vi "readFrequencySweep(sub).vi"(0 "resourcein":refnum<visa-resource-name>, 1 "Command":dbl, 2 "Commandprefix":string="R0003", 3 "errorin":errorcluster, 4 "Numeric":i32) -> (5 "resourceout":refnum<visa-resource-name>, 6 "Array":string[](array[string]), 7 "errorout":errorcluster)   [LabVIEW 2015]
panel:
  out "output 2":string
  out "output 1":dbl
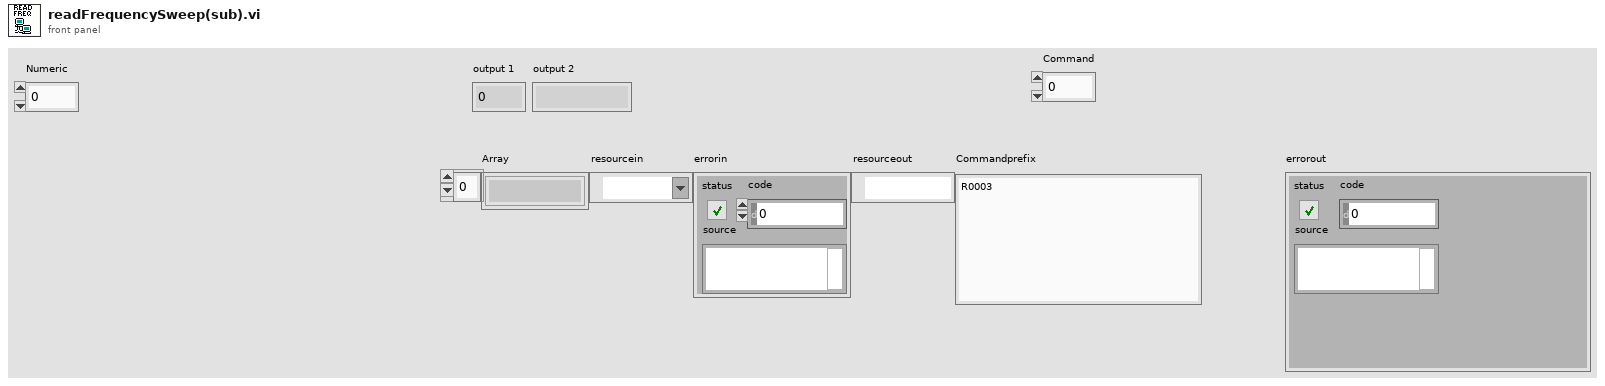
[diagram p1: front panel]
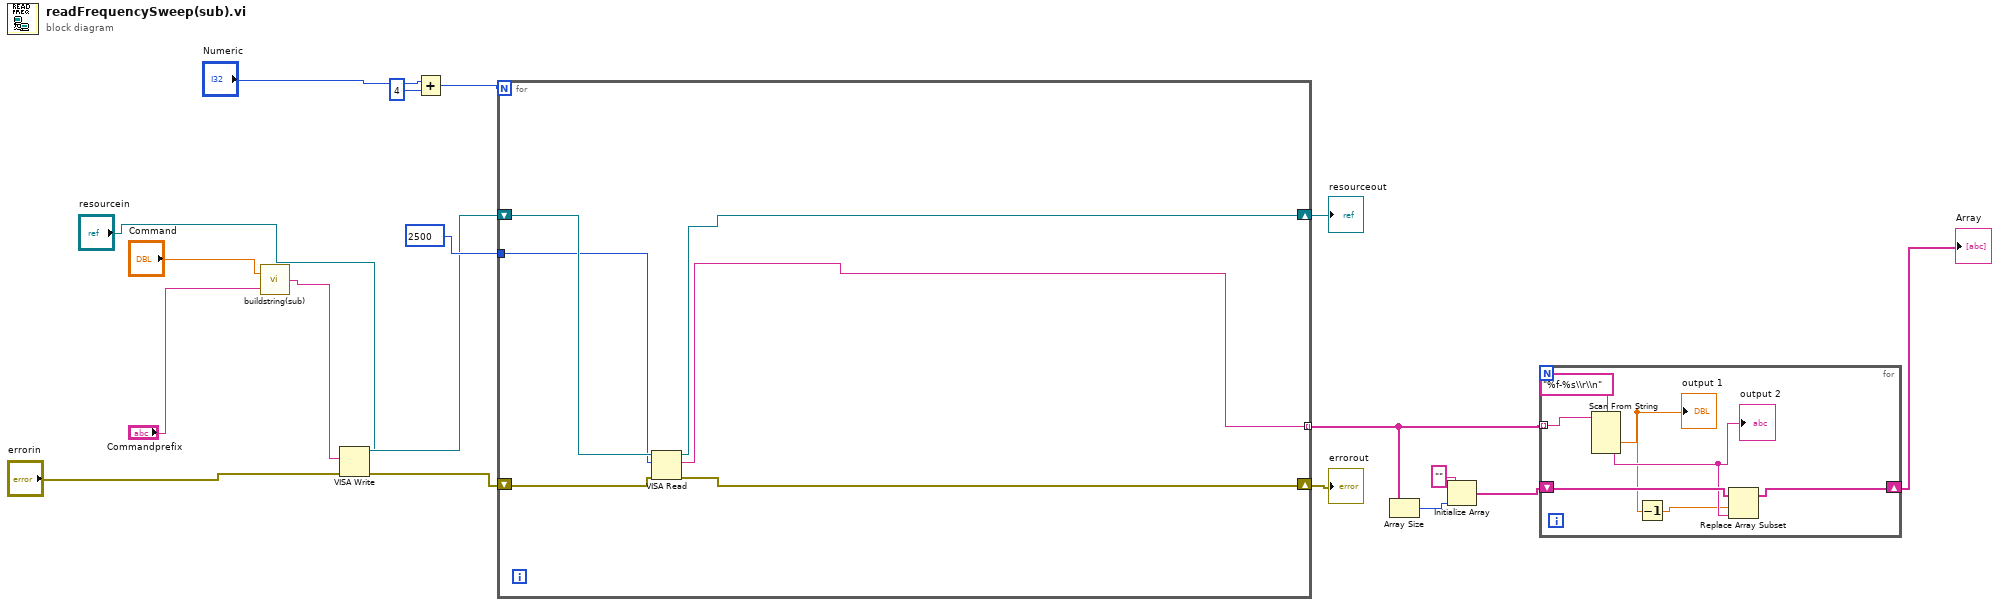
[diagram p0: block diagram]
diagram:
  n1 = call "buildstring(sub).vi"("Prefix"="Commandprefix", "Command"="Command") -> ("Commandstring"=w15:string)
  n2 = VISA Write(VISA resource name="resourcein", write buffer=w15, error in (no error)="errorin") -> (VISA resource name out=w10:refnum<visa-resource-name>, error out=w11:errorcluster)  [unwired: 1 out]
  n3 = Add(x="Numeric", y=4) -> (x+y=w2:i32)
  n4 = for {
    N: w2 -> [_]
    tunnel: u32 2500 ("byte count") -> [w20]
    shift-right: [w22] -> w18
    shift-left: w11 -> [w23]
    shift-right: [w21] -> w17
    shift-left: w10 -> [w24]
    tunnel: [w19] -> w8 mode=indexing
    n5 = VISA Read(VISA resource name=w24, byte count=w20, error in (no error)=w23) -> (VISA resource name out=w21:refnum<visa-resource-name>, read buffer=w19:string, error out=w22:errorcluster)  [unwired: 1 out]
  }
  "errorout" <- w18
  "resourceout" <- w17
  n6 = Array Size(array=w8) -> (size(s)=w4:i32)
  n7 = Initialize Array("" ("format string"), w4) -> (w6:string[])
  n8 = for {
    tunnel: w8 -> [w31] mode=indexing
    shift-right: [w28] -> w5
    shift-left: w6 -> [w29]
    n9 = Scan From String(format string="%f-%s\\r\\n", input string=w31) -> (output 1=w25:dbl, output 2=w27:string)  [unwired: 4 in, 3 out]
    "output 1" <- w25
    "output 2" <- w27
    n10 = Decrement(x=w25) -> (x-1=w26:dbl)
    n11 = Replace Array Subset(array=w29, new element=w27, index=w26) -> (w28:string[])
  }
  "Array" <- w5
